vi "Spaghetti.vi"(8 "error in (no error)":errorcluster, 11 "Tamagotchi Full Actor in":refnum<class "Tamagotchi Full Actor.lvclass">) -> (0 "error out":errorcluster, 3 "Tamagotchi Full Actor out":refnum<class "Tamagotchi Full Actor.lvclass">)   [LabVIEW 2026, in "Tamagotchi Full Actor.lvclass"]
uses:
  Tamagotchi Full Actor.lvclass
  Tamagotchi Full Actor.lvclass/Tamagotchi Full Actor.ctl
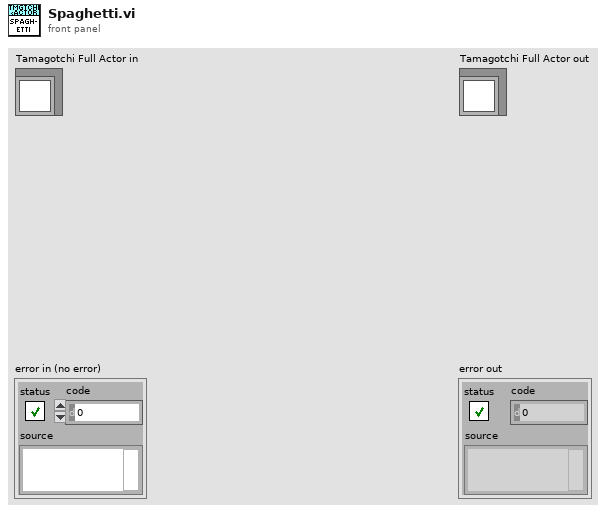
[diagram p1: front panel]
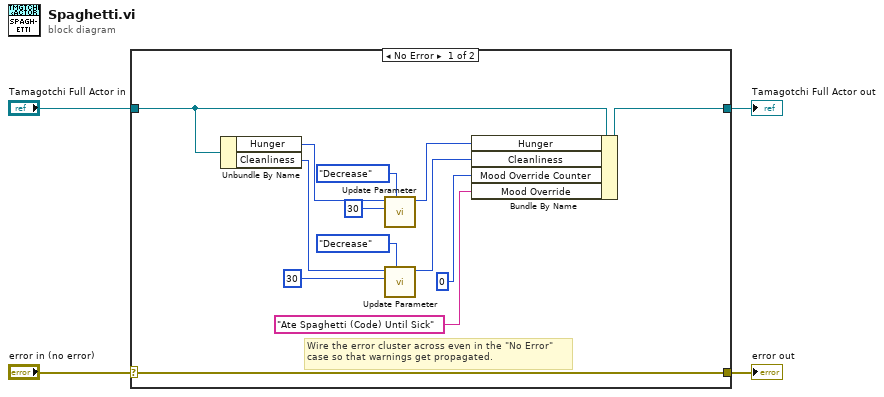
[diagram p0: block diagram]
diagram:
  n1 = case shown="No Error" "error in (no error)" {
    selector: "error in (no error)" -> [w17 w19]
    tunnel: [w17 w19] -> w3
    tunnel: [w5 w18] -> w1
    tunnel: "Tamagotchi Full Actor in" -> [w6 w18]
    frame No Error {
      # "Wire the error cluster across even in the \"No Error\"\ncase so that warnings get propagated."
      n2 = Unbundle By Name(w6) -> ("Hunger"=w9:i16, "Cleanliness"=w15:i16)
      n3 = call "Update Parameter.vi"("Action"=enum16{"Increase", "Decrease"}."Decrease", "Modifier"=i16 30 ("y"), "Parameter"=w9) -> ("New Value"=w10:i16)  [unwired: 8 in]
      n4 = call "Update Parameter.vi"("Action"=enum16{"Increase", "Decrease"}."Decrease", "Modifier"=i16 30 ("y"), "Parameter"=w15) -> ("New Value"=w16:i16)  [unwired: 8 in]
      n5 = Bundle By Name(cluster=w6, "Hunger"=w10, "Cleanliness"=w16, "Mood Override Counter"=u32 0, "Mood Override"="Ate Spaghetti (Code) Until Sick") -> (w5:refnum<class "Tamagotchi Full Actor.lvclass">)
    }
    frame Error {
    }
  }
  "error out" <- w3
  "Tamagotchi Full Actor out" <- w1
